vi "phy_dpsk_mod.vi"(8 "type":enum16{"binary", "quadrature"}(ring), 11 "input bits":i8[](array[numeric])) -> (0 "last phase":dbl, 3 "dpsk":cdb[](array[numeric]))   [LabVIEW 2014]
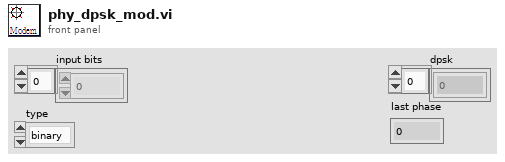
[diagram p1: front panel]
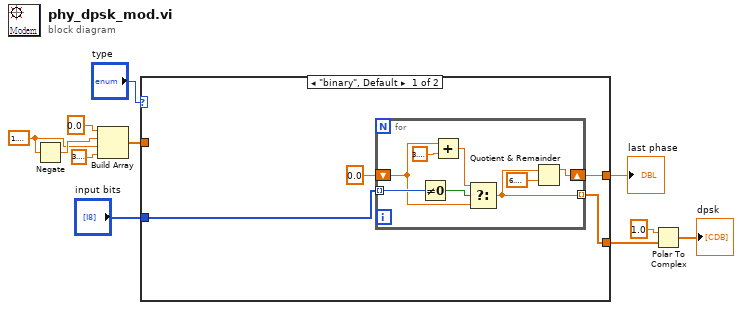
[diagram p0: block diagram]
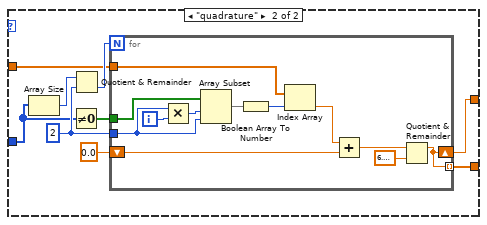
[diagram p2: hidden frame]
diagram:
  w1 = 1.5707963267948966
  n1 = Negate(x=w1) -> (-x=w2:dbl)
  n2 = Build Array(0.0, w2, w1, 3.141592653589793) -> (w7:dbl[])
  n3 = case shown="\"binary\", Default" "type" {
    tunnel: "input bits" -> [w14 w29]
    tunnel: [w13 w24] -> w5
    tunnel: [w12 w26] -> w10
    tunnel: w7 -> [_ w25]
    frame "binary", Default {
      n4 = for {
        shift-right: [w17] -> w12
        shift-left: 0.0 -> [w20]
        tunnel: w14 -> [w23] mode=indexing
        tunnel: [w16] -> w13 mode=indexing
        n5 = Not Equal To 0?(x=w23) -> (x != 0?=w22:bool)
        n6 = Add(x=w20, y=3.141592653589793) -> (x+y=w19:dbl)
        n7 = Select(t=w19, s=w22, f=w20) -> (s? t:f=w16:dbl)
        n8 = Quotient & Remainder(x=w16, y=6.283185307179586) -> (x-y*floor(x/y)=w17:dbl)  [unwired: 1 out]
      }
    }
    frame "quadrature" {
      w30 = 2 ("y")
      n9 = Array Size(array=w29) -> (size(s)=w32:i32)
      n10 = Not Equal To 0?(x=w29) -> (x != 0?=w28:bool[])
      n11 = Quotient & Remainder(x=w32, y=w30) -> (floor(x/y)=w31:i32)  [unwired: 1 out]
      n12 = for {
        N: w31 -> [_]
        tunnel: w28 -> [w41]
        tunnel: w30 -> [w42]
        shift-right: [w33] -> w26
        shift-left: 0.0 -> [w36]
        tunnel: w25 -> [w39]
        tunnel: [w33] -> w24 mode=indexing
        i -> [w44]
        n13 = Multiply(x=w42, y=w44) -> (x*y=w43:i32)
        n14 = Array Subset(array=w41, index=w43, length=w42) -> (w40:bool[])
        n15 = Boolean Array To Number(Boolean array=w40) -> (number=w38:u32)
        n16 = Index Array(array=w39, index=w38) -> (element=w37:dbl)
        n17 = Add(x=w37, y=w36) -> (x+y=w35:dbl)
        n18 = Quotient & Remainder(x=w35, y=6.283185307179586) -> (x-y*floor(x/y)=w33:dbl)  [unwired: 1 out]
      }
    }
  }
  "last phase" <- w10
  n19 = Polar To Complex(1:w5, 2:1.0) -> (0:→"dpsk":cdb[])
